vi "RemoveChars.vi"(0 "String":string, 5 "Max chars to remove":i32=-1 caption="Max chars to remove (-1 = all)", 7 "Chars to remove":string[](array[string]) caption="Chars to remove (empty = any)") -> (4 "Shortened string":string)   [LabVIEW 2017, in "GPString.lvlib"]
doc: "Removes a number of characters from <B>String</B> and returns the result in <B>Shortened string</B>.\n\nThis VI starts at the front of <B>String</B>, removing character by character as long as the encountered character is found in the <B>Chars to remove</B> array with an upper limit of <B>Max chars to remove</B>.\n\nYou can leave <B>Max chars to remove</B> at -1 to have no upper limit, letting this VI remove characters until it encounters one that isn't in the <B>Chars to remove</B> array.\n\nYou can leave the <B>Chars to remove</B> array empty to remove any character value only stopping when <B>Max chars to remove</B> has been reached.\n\nThis VI is inlined.\n\nSteen Schmidt\nGPower\n25/9 2015"
uses:
  GPString.lvlib
  Numeric/GPNumeric.lvlib
panel:
  # "Copyright © 2015\nGPower\nSee enclosed license file for terms and conditions"
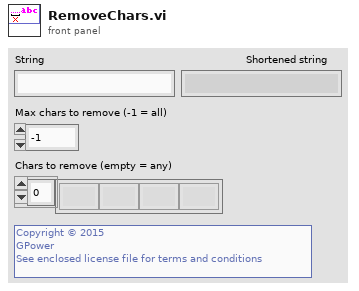
[diagram p1: front panel]
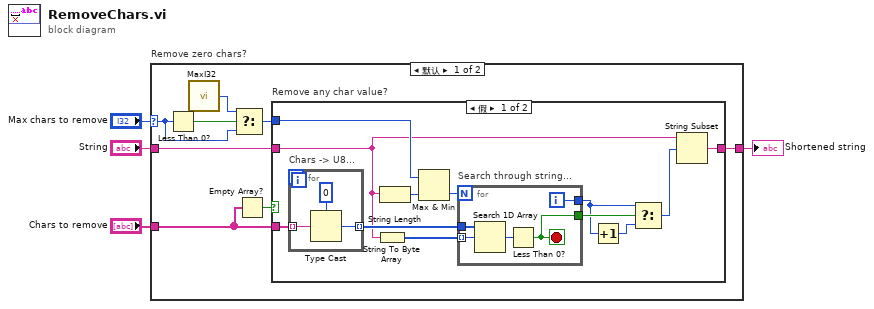
[diagram p0: block diagram]
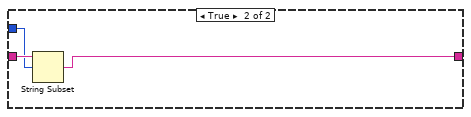
[diagram p2: hidden frame]
diagram:
  n1 = case "Remove zero chars?" shown="默认" "Max chars to remove" {
    selector: "Max chars to remove" -> [w6 _]
    tunnel: "Chars to remove" -> [w10 _]
    tunnel: "String" -> [w12 w36]
    tunnel: [w11 w36] -> w2
    frame Default {
      n2 = Less Than 0?(x=w6) -> (x < 0?=w8:bool)
      n3 = call "MaxI32.vi"() -> ("Maximum value"=w7:i32)
      n4 = Select(t=w7, s=w8, f=w6) -> (s? t:f=w5:i32)
      n5 = Empty Array?(array=w10) -> (empty?=w9:bool)
      n6 = case "Remove any char value?" shown="假" w9 {
        tunnel: w10 -> [w24 _]
        tunnel: w5 -> [w21 w34]
        tunnel: w12 -> [w19 w35]
        tunnel: [w18 w33] -> w11
        frame False {
          n7 = for "Chars -> U8..." {
            tunnel: w24 -> [w27] mode=indexing
            tunnel: [w26] -> w23 mode=indexing
            n8 = Type Cast(type=u8 0, x=w27) -> (*(type *) &x=w26:u8)
          }
          n9 = String To Byte Array(string=w19) -> (unsigned byte array=w22:u8[])
          n10 = String Length(string=w19) -> (length=w20:i32)
          n11 = Max & Min(x=w21, y=w20) -> (min(x,y)=w17:i32)  [unwired: 1 out]
          n12 = for "Search through string..." {
            N: w17 -> [_]
            tunnel: w22 -> [w31] mode=indexing
            tunnel: w23 -> [w32]
            tunnel: [w29] -> w15
            tunnel: [w28] -> w16
            i -> [w29]
            stop <- w28 stop-if-true
            n13 = Search 1D Array(1D array=w32, element=w31) -> (index of element=w30:i32)  [unwired: 1 in]
            n14 = Less Than 0?(x=w30) -> (x < 0?=w28:bool)
          }
          n15 = Increment(x=w15) -> (x+1=w14:i32)
          n16 = Select(t=w15, s=w16, f=w14) -> (s? t:f=w13:i32)
          n17 = String Subset(string=w19, offset (0)=w13) -> (substring=w18:string)  [unwired: 1 in]
        }
        frame True {
          n18 = String Subset(string=w35, offset (0)=w34) -> (substring=w33:string)  [unwired: 1 in]
        }
      }
    }
    frame 0 {
    }
  }
  "Shortened string" <- w2
